vi "CalibMeasure.vi"(8 "error in (no error)":errorcluster, 10 "calibration_id":i32, 11 "ByteGSAPIBase in":refnum<class "ByteGSAPIBase.lvclass">) -> (0 "error out":errorcluster, 2 "Cluster":T1={"strumento_riferimento"={"id"=0, "nome"=""}, "controls"=[], "temperatura"=25.0, "umidita"=80.0} {"umidita" format="%.1g"; "temperatura" format="%.1g"; "controls"."incertezza" format="%.1g"; "controls"."deviazione_standard" format="%.1g"; "controls"."mpe_min" format="%.1g"; "controls"."mpe_max" format="%.1g"; "controls"."riferimento_obiettivo" format="%.1g"}, 3 "ByteGSAPIBase out":refnum<class "ByteGSAPIBase.lvclass">)   [LabVIEW 2019, in "ByteGSWebAPI.lvlib" / "ByteGSAPIBase.lvclass"]
uses:
  ByteGSAPIBase.lvclass
  BodyCalibrazioneMisure.ctl
  <vilib>/Bytelabs/ByteREST/ByteRESTClass/ByteRESTBase/HTTP/Status_Code.ctl
  ByteGSAPIBase.lvclass/ByteGSAPIBase.ctl
  <vilib>/Bytelabs/ByteREST/ByteRESTClass/ByteRESTBase/RESTBase.lvclass
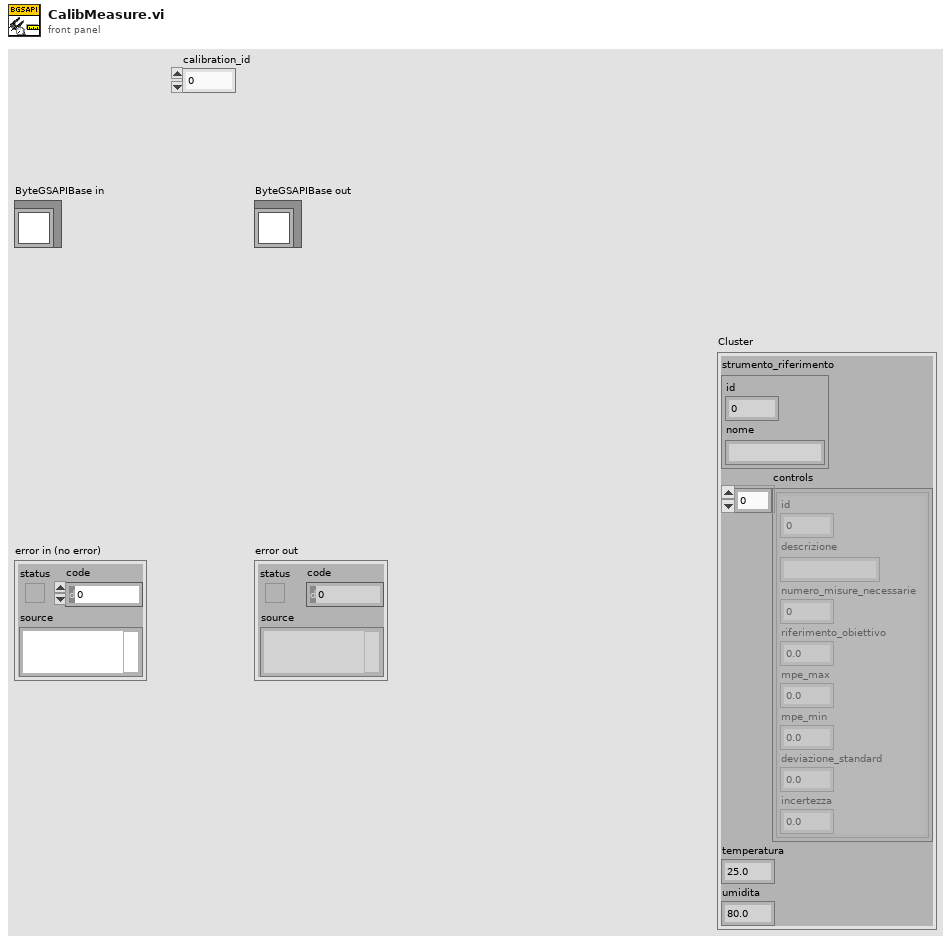
[diagram p1: front panel]
types:
  T1 = typedef "BodyCalibrazioneMisure.ctl" = cluster{"strumento_riferimento":cluster{"id":u16, "nome":string}, "controls":cluster{"id":u16, "descrizione":string, "numero_misure_necessarie":u16, "riferimento_obiettivo":dbl, "mpe_max":dbl, "mpe_min":dbl, "deviazione_standard":dbl, "incertezza":dbl}[], "temperatura":dbl, "umidita":dbl}
  T2 = typedef "ByteREST.lvlib/RESTBase.lvclass/Status_Code.ctl" = u16
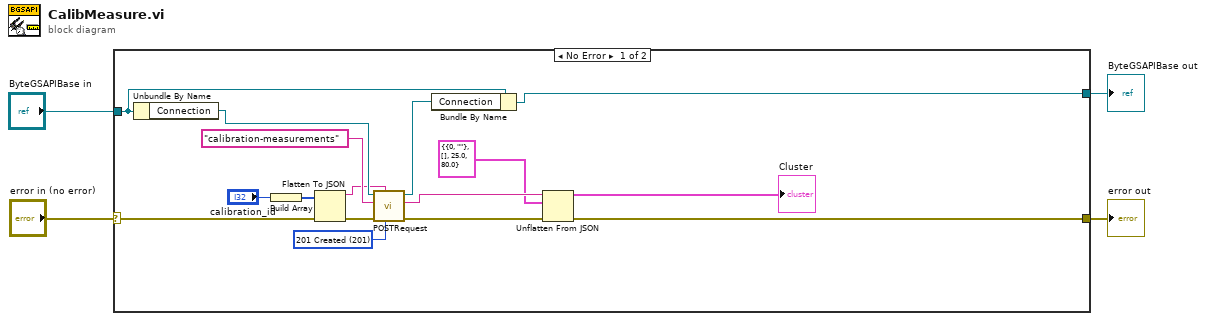
[diagram p0: block diagram]
diagram:
  n1 = case shown="No Error" "error in (no error)" {
    selector: "error in (no error)" -> [w15 w22]
    tunnel: [w5 w22] -> w3
    tunnel: [w18 w21] -> w1
    tunnel: "ByteGSAPIBase in" -> [w20 w21]
    frame No Error {
      w12 = T2 201 items=["200 OK"=200, "201 Created"=201, "400 Bad Request"=400, "401 Unauthorized"=401, "403 Forbidden"=403, "404 Not Found"=404, "405 Method Not Allowed"=405, "406 Not Acceptable"=406, "500 Internal Server Error"=500] ("expected response")
      n2 = Unbundle By Name(w20) -> ("Connection"=w19:refnum<class "RESTBase.lvclass">)
      n3 = Build Array("calibration_id") -> (w8:i32[])
      n4 = Flatten To JSON(anything=w8, error in (no error)=w15) -> (JSON string=w10:string, 11:w11:errorcluster)  [unwired: 1 in]
      n5 = call-dynamic "POSTRequest.vi"("expected response"=w12, "Body in"=w10, "error in (no error)"=w11, "Request"="calibration-measurements", "ByteRESTBase in"=w19) -> ("error out"=w13:errorcluster, "Body"=w14:string, "ByteRESTBase out"=w17:refnum<class "RESTBase.lvclass">)  [unwired: 3 in, 1 out]
      n6 = Bundle By Name(cluster=w20, "Connection"=w17) -> (w18:refnum<class "ByteGSAPIBase.lvclass">)
      n7 = Unflatten From JSON(JSON string=w14, type and defaults=T1 {"strumento_riferimento"={"id"=0, "nome"=""}, "controls"=[], "temperatura"=25.0, "umidita"=80.0} ("Cluster 2"), error in (no error)=w13) -> (value=→"Cluster":T1, error out=w5:errorcluster)  [unwired: 4 in]
    }
    frame Error {
    }
  }
  "error out" <- w3
  "ByteGSAPIBase out" <- w1
